vi "WAV_Query.vi"(0 "System no.":i32=1 min=1 max=4 step=1, 2 "Axes to query":string[](array[string]), 3 "Parameter no.":i32[](array[numeric]), 5 "error in":errorcluster) -> (14 "WAV Parameter value":dbl[](array[numeric]) format="%.6f", 19 "error out":errorcluster)   [LabVIEW 2020]
doc: "Returns waveform parameter values for queried axes and parameter numbers. \n\nAll systems: Affected axis is identical with wave table number. The following parameter number is valid: \n- 1: Number of waveform points for currently defined wave"
uses:
  Global1.vi
panel:
  # "Returns waveform parameter values for queried axes and parameter numbers."
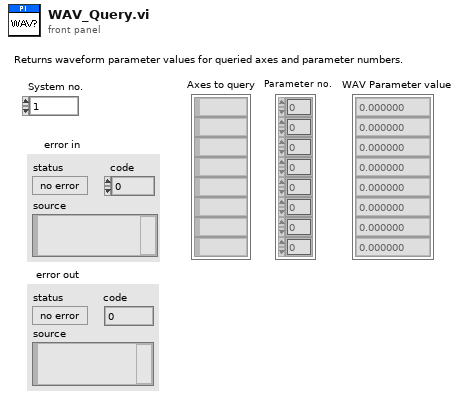
[diagram p1: front panel]
types:
  T1 = typedef "Syntax.ctl" = enum16{"GCS 1.0", "GCS 2.0", "GCS 3.0"}
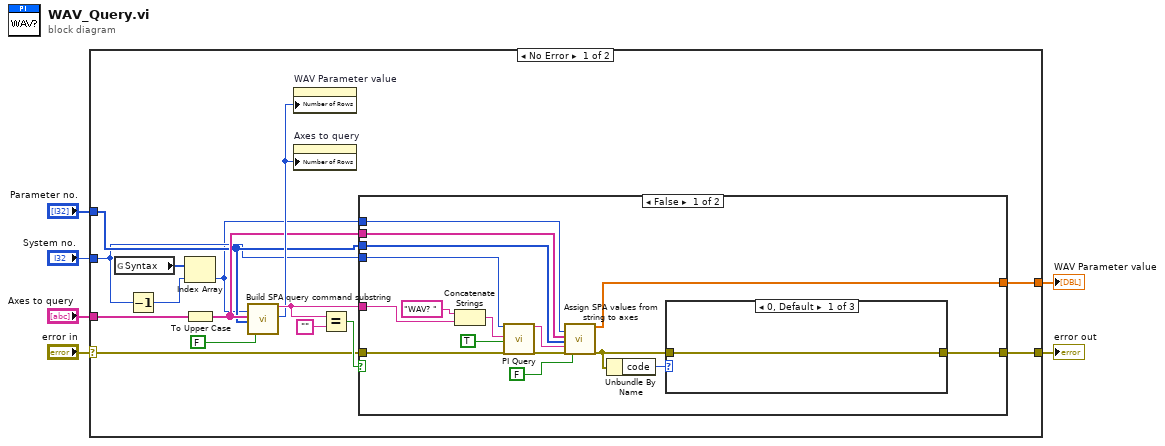
[diagram p0: block diagram]
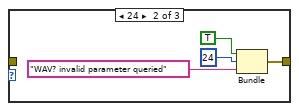
[diagram p2: hidden frame]
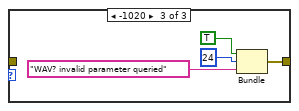
[diagram p3: hidden frame]
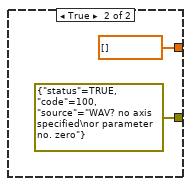
[diagram p4: hidden frame]
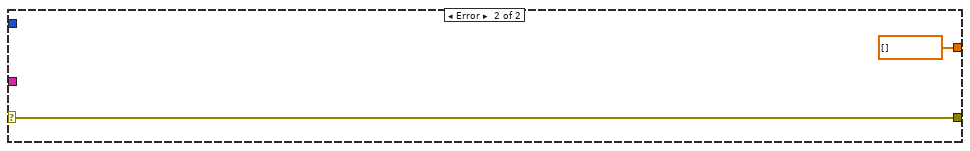
[diagram p5: hidden frame]
diagram:
  n1 = case shown="No Error" "error in" {
    selector: "error in" -> [w7 w49]
    tunnel: "Axes to query" -> [w21 _]
    tunnel: "System no." -> [w10 _]
    tunnel: "Parameter no." -> [w16 _]
    tunnel: [w15 w49] -> w3
    tunnel: [w13 dbl[] [] ("Parameter values")] -> w2
    frame No Error {
      n2 = global read "Global1.vi" "Syntax"() -> (w11:T1[])
      n3 = Decrement(x=w10) -> (x-1=w12:i32)
      n4 = Index Array(array=w11, index=w12) -> (element=w9:T1)
      n5 = To Upper Case(1:w21) -> (0:w17:string[])
      n6 = call "Build SPA query command substring.vi"("Syntax"=w9, "Axes to query"=w17, "Parameter number"=w16, "Parameter no. format \n(Decimal: FALSE)"=FALSE ("Parameter no. format \n(Decimal: FALSE)")) -> ("Command substring"=w19:string, "Number of rows"=w18:u32)  [unwired: 3 in, 11 out]
      n7 = property on="WAV Parameter value" class="Arr (strict)"("Number of Rows"=w18) -> ()  [unwired: 2 in, 2 out]
      n8 = property on="Axes to query" class="Arr (strict)"("Number of Rows"=w18) -> ()  [unwired: 2 in, 2 out]
      n9 = Equal?(x=w19, y="" ("x")) -> (x = y?=w14:bool)
      n10 = case shown="False" w14 {
        tunnel: w7 -> [w30 _]
        tunnel: w19 -> [w34 _]
        tunnel: w17 -> [w33 _]
        tunnel: w10 -> [w29 _]
        tunnel: w16 -> [w32 _]
        tunnel: [w24 errorcluster {"status"=TRUE, "code"=100, "source"="WAV? no axis specified\nor parameter no. zero"} ("error out")] -> w15
        tunnel: [w31 dbl[] [] ("Parameter values")] -> w13
        tunnel: w9 -> [w27 _]
        frame False {
          n11 = Concatenate Strings("WAV? ", w34) -> (w35:string)
          n12 = call "PI Query.vi"("System no."=w29, "String to send"=w35, "Attach termination char.?"=TRUE ("Attach Linefeed?"), "error in"=w30) -> ("String read"=w25:string, "error out"=w26:errorcluster)  [unwired: 3 in, 11 out]
          n13 = call "Assign SPA values from string to axes.vi"("Syntax"=w27, "Queried axes"=w33, "Parameter no."=w32, "Input string"=w25, "error in"=w26, "Parameter no. format \n(Decimal: FALSE)"=FALSE ("Parameter no. format \n(Decimal: FALSE)")) -> ("Parameter values"=w31:dbl[], "error out"=w22:errorcluster)  [unwired: 2 in, 10 out]
          n14 = Unbundle By Name(w22) -> ("code"=w23:i32)
          n15 = case shown="0, Default" w23 {
            tunnel: [w38 w39 w43] -> w24
            tunnel: w22 -> [w38 _ _]
            frame 0, Default {
            }
            frame 24 {
              n16 = Bundle(TRUE, 24, "WAV? invalid parameter queried") -> (w39:errorcluster)  [unwired: 1 out]
            }
            frame -1020 {
              n17 = Bundle(TRUE, 24, "WAV? invalid parameter queried") -> (w43:errorcluster)  [unwired: 1 out]
            }
          }
        }
        frame True {
        }
      }
    }
    frame Error {
    }
  }
  "error out" <- w3
  "WAV Parameter value" <- w2
